vi "Main.GUI.vi"() -> ()   [LabVIEW 2015, in "Main.GUI.lvlib"]
uses:
  Main.GUI.lvlib
  Types/Multihead.StateVariables.ctl
  Types/TestStandGUI.Refs.ctl
  <vilib>/NI Veristand/Execution/Workspace/WorkspaceAPI.ctl
  <vilib>/NI Veristand/Execution/Workspace/SystemStateEventRef.ctl
  <vilib>/NI Veristand/Execution/Workspace/Target State Info.ctl
  <vilib>/NI Veristand/Execution/Workspace/Target State.ctl
  Execution GUI/Types/Execute.UserEventRefs.ctl
  <vilib>/NI Veristand/Execution/Workspace/SystemStateRegEventRef.ctl
  Analysis GUI/Types/Analysis.GUI.Parameters.ctl
  NationalInstruments.VeriStand
  <vilib>/NI/AMC/Read Termination Message.vi
  <vilib>/NI/AMC/Update Message Routing Info.vi
  <vilib>/NI/AMC/Create Multiple Messages.vi
  <vilib>/NI/AMC/Create Single Message.vi
  <vilib>/NI/AMC/Globals.vi
  <vilib>/NI/AMC/Send Message.vi
  <vilib>/NI Veristand/Execution/Workspace/NI VeriStand - Set Multiple Channel Values.vi
  <vilib>/NI/AMC/Queue Registry.vi
  <vilib>/NI/AMC/AMC.lvlib
  <vilib>/NI Veristand/Execution/Workspace/NI_VS Workspace ExecutionAPI.lvlib
  Execution GUI/Station.Execution.lvlib
  Analysis GUI/Analysis.lvlib
  NationalInstruments.VeriStand.ClientAPI
panel:
  in  "NIVS.Workspace Event":refnum<event-registration>
  in  "Application Manager":refnum<k7>(container)
  in  "SequenceFileView Manager":refnum<k7>(container)
  in  "ExecutionView Manager":refnum<k7>(container)
  in  "Tab Control":enum32{"TestStand", "GUIs"}(tab)
  in  "Entry Point 2 Button":refnum<k7>(container)
  in  "Open Sequence File Button":refnum<k7>(container)
  in  "Execution View":refnum<k7>(container)
  in  "Stop":bool
  out "Path":path
  in  "NIVS.Gateway IP Address":string="localhost"
  in  "Tree":string(tree)
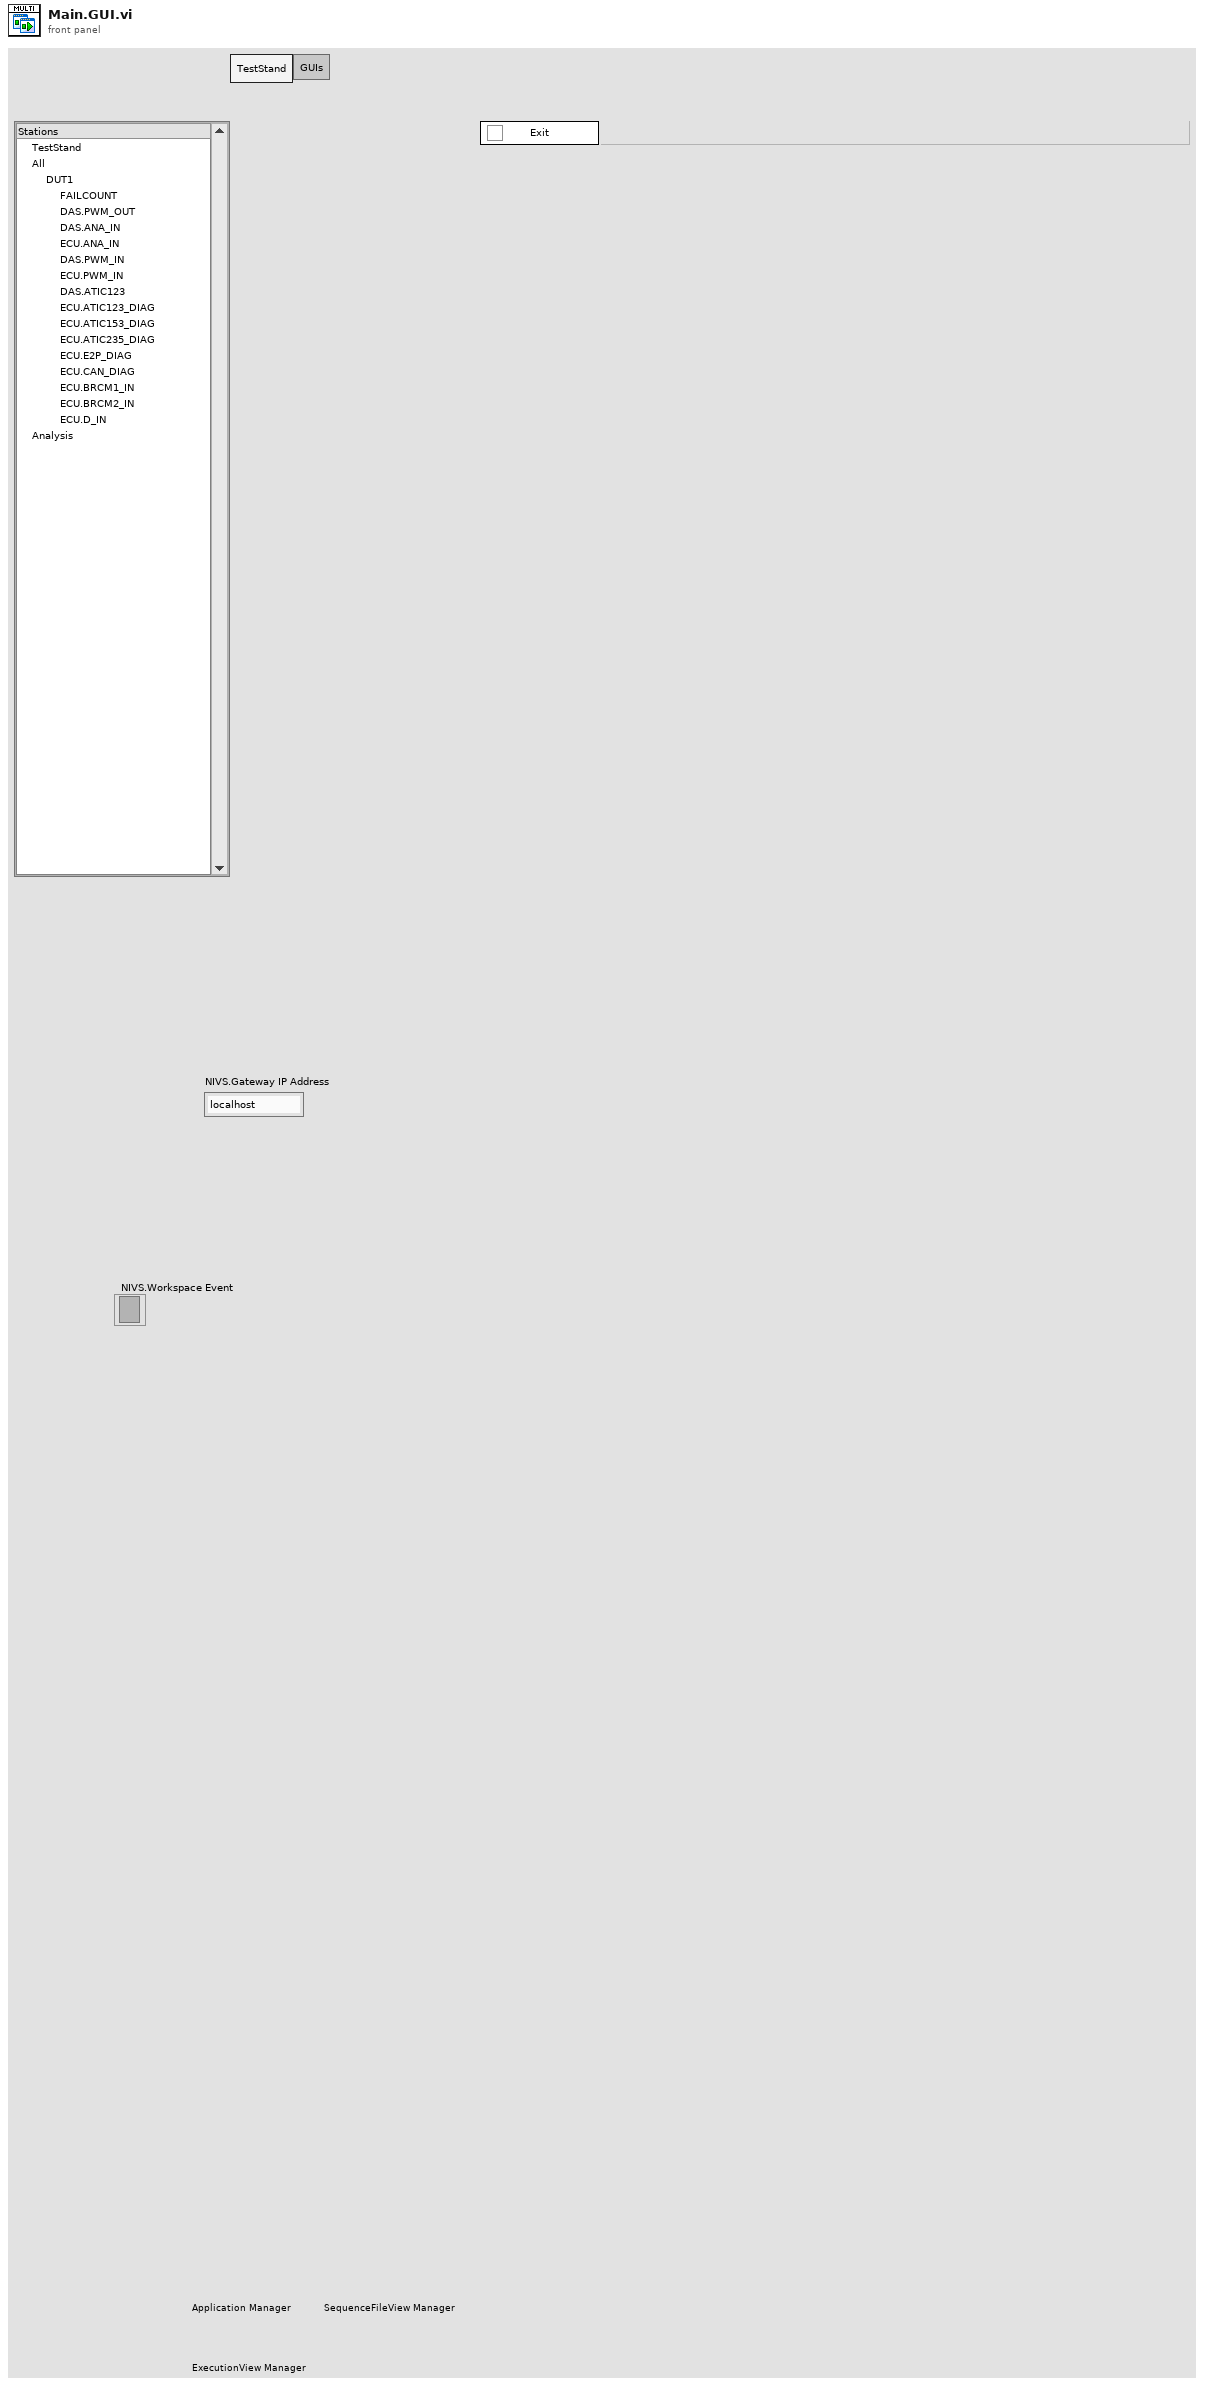
[diagram p1: front panel]
types:
  T1 = typedef "Main.GUI.lvlib/Multihead.StateVariables.ctl" = cluster{"DUTs.Name":string[], "Pages.Name":string[], "Pages.Ref":refnum<vi>[], "TS.UI":T2, "TS.Running":bool, "TS.Abort":bool, "NIVS.GatewayIPAddress":string, "NIVS.WorkspaceManager":T3, "NIVS.Open":bool, "NIVS.Deployed":bool, "NIVS.SystemStateRefs":T4, "NIVS.Events":T5, "UI.Tree":refnum<vi>, "UI.Path":refnum<vi>, "UI.Stop":refnum<vi>, "UI.Tab":refnum<vi>}
  T2 = typedef "Main.GUI.lvlib/TestStandGUI.Refs.ctl" = cluster{"References":cluster{"Event Callback":refnum<k27>, "Quit Application Event":refnum<user-event>, "Events":refnum<event-registration>, "Top level VI":refnum<vi>, "TestStand Engine":refnum<k7>, "Start Application Event":refnum<user-event>, "Stop Application Event":refnum<user-event>}, "Managers":cluster{"Application Manager":refnum<k7>, "SequenceFileView Manager":refnum<k7>, "ExecutionView Manager":refnum<k7>}, "Controls":cluster{"Execution View":refnum<k7>, "Run Button":refnum<k7>, "Open Button":refnum<k7>}}
  T3 = typedef "NI_VS Workspace ExecutionAPI.lvlib/WorkspaceAPI.ctl" = refnum<k24>
  T4 = typedef "NI_VS Workspace ExecutionAPI.lvlib/SystemStateEventRef.ctl" = cluster{"CustDatRef":refnum<user-event>, "EvtRef":refnum<k27>, "Target State User Event":refnum<user-event>}
  T5 = typedef "Station.Execution.lvlib/Execute.UserEventRefs.ctl" = cluster{"SystemChangeEvent":T6, "WorkspaceEvent":refnum<event-registration>}
  T6 = typedef "NI_VS Workspace ExecutionAPI.lvlib/SystemStateRegEventRef.ctl" = refnum<event-registration>
  T7 = typedef "AMC.lvlib/Message Queue.ctl" = refnum<queue>
  T8 = typedef "Analysis.lvlib/Analysis.GUI.Parameters.ctl" = cluster{"Results Path":path, "Temp Path":path, "Remote Path":path, "Analysis VIs":path[], "Report Passed?":bool, "Group Channels?":bool}
  T9 = cluster{"SystemChangeEvent":T6, "WorkspaceEvent":refnum<event-registration>, "Events":refnum<event-registration>}
  T10 = typedef "NI_VS Workspace ExecutionAPI.lvlib/SystemState.ctl" = u8
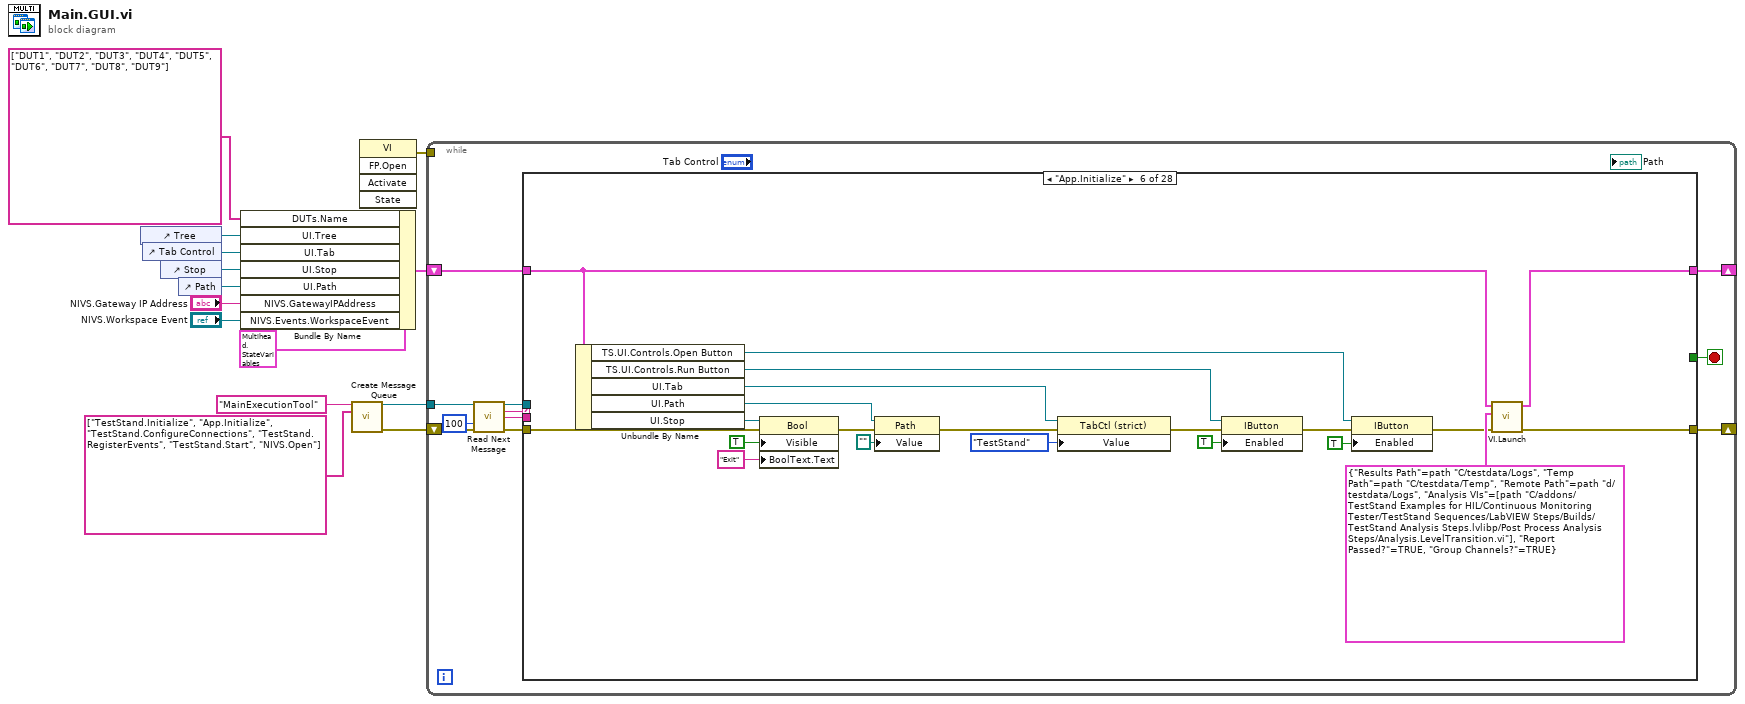
[diagram p0: block diagram]
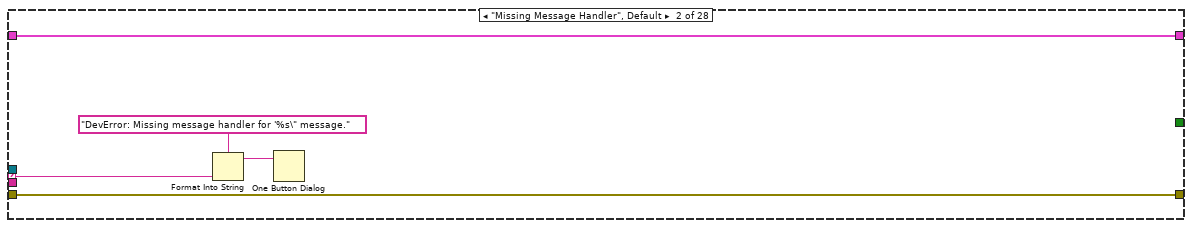
[diagram p3: hidden frame]
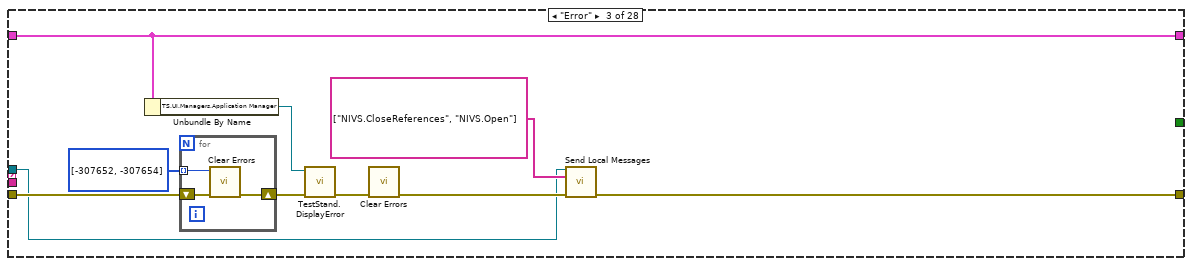
[diagram p4: hidden frame]
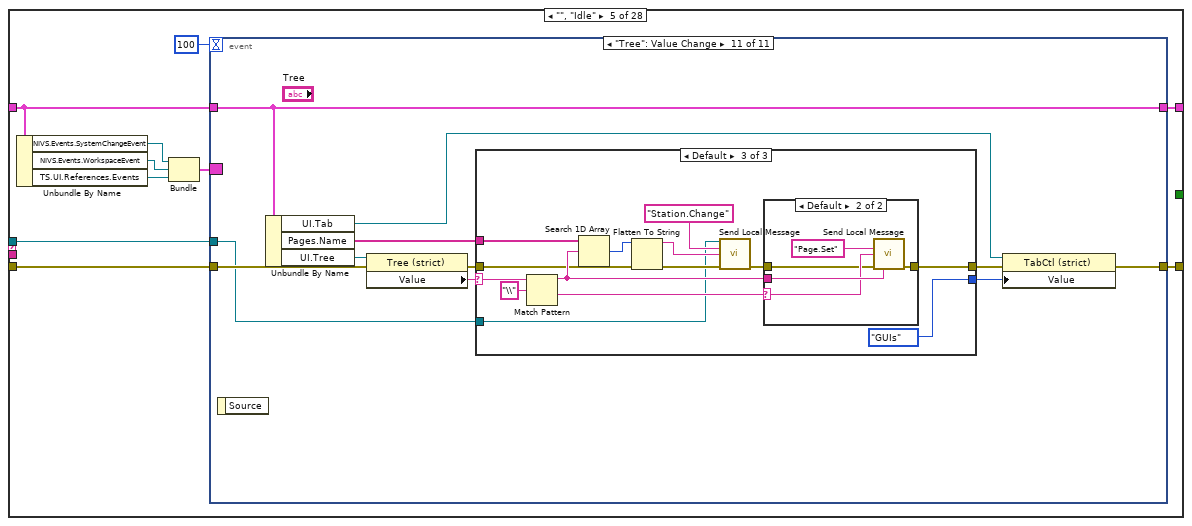
[diagram p6: hidden frame]
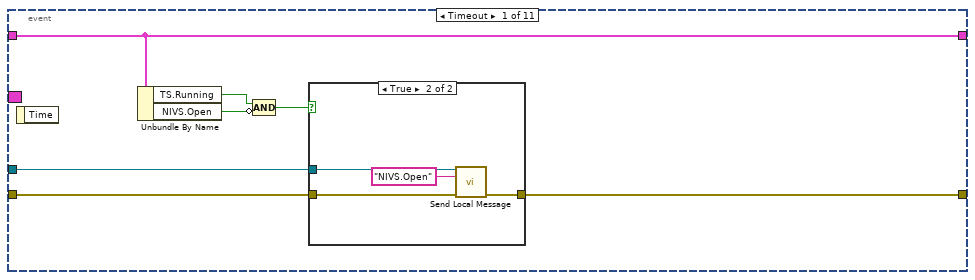
[diagram p7: hidden frame]
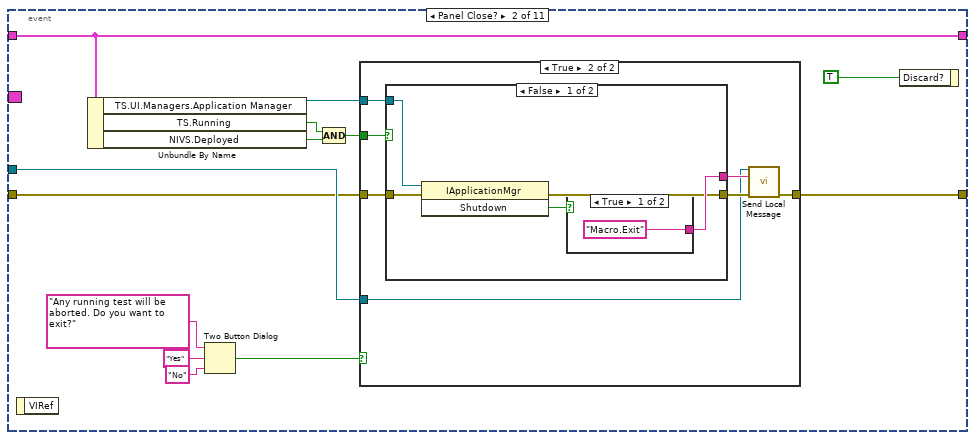
[diagram p9: hidden frame]
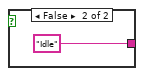
[diagram p11: hidden frame]
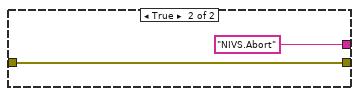
[diagram p12: hidden frame]
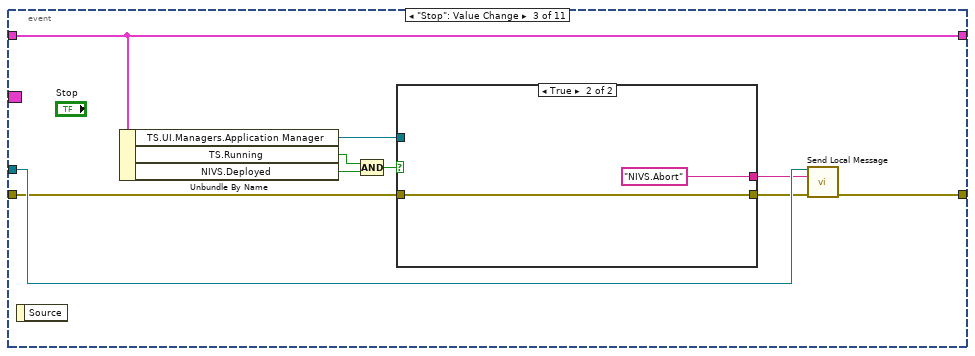
[diagram p13: hidden frame]
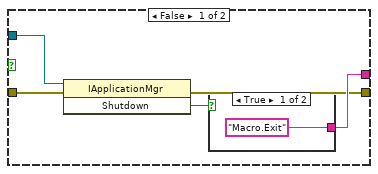
[diagram p14: hidden frame]
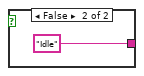
[diagram p15: hidden frame]
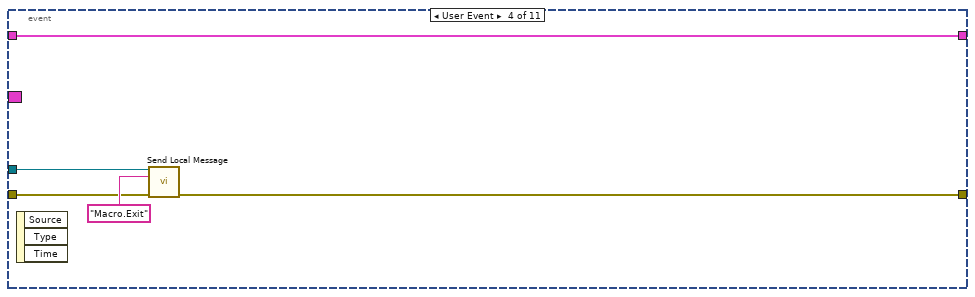
[diagram p16: hidden frame]
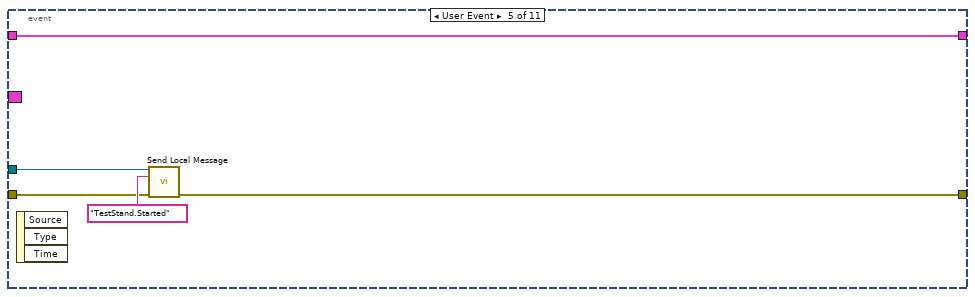
[diagram p17: hidden frame]
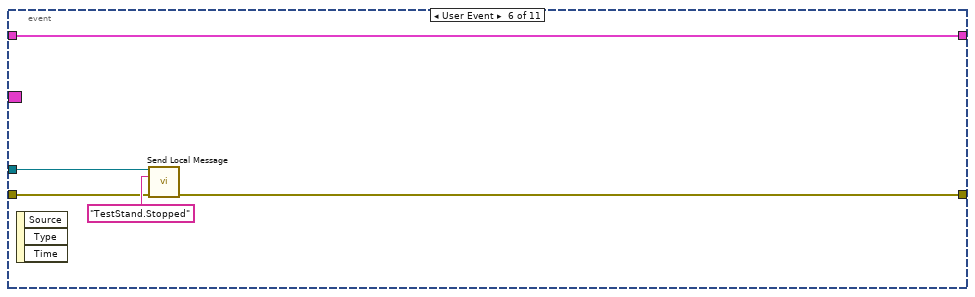
[diagram p18: hidden frame]
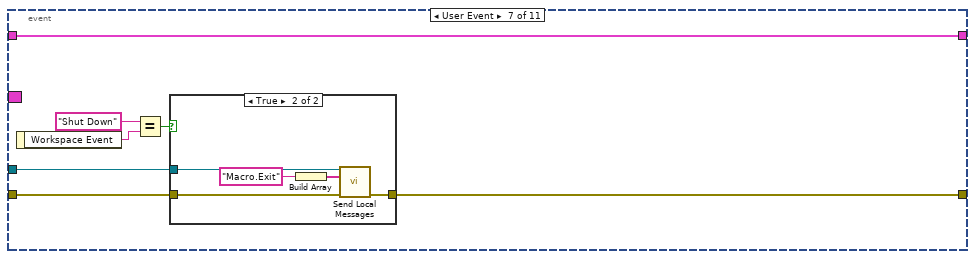
[diagram p19: hidden frame]
diagram:
  n1 = control-ref of="Tree"() -> (w13:refnum<vi>)
  n2 = control-ref of="Tab Control"() -> (w8:refnum<vi>)
  n3 = control-ref of="Stop"() -> (w7:refnum<vi>)
  n4 = control-ref of="Path"() -> (w1:refnum<vi>)
  n5 = Bundle By Name(cluster=T1 {"DUTs.Name"=[], "Pages.Name"=[], "Pages.Ref"=[], "TS.UI"={"References"={"Event Callback"=refnum, "Quit Application Event"=refnum, "Events"=refnum, "Top level VI"=refnum, "TestStand Engine"=refnum, "Start Application Event"=refnum, "Stop Application Event"=refnum}, "Managers"={"Application Manager"=refnum, "SequenceFileView Manager"=refnum, "ExecutionView Manager"=refnum}, "Controls"={"Execution View"=refnum, "Run Button"=refnum, "Open Button"=refnum}}, "TS.Running"=FALSE, "TS.Abort"=FALSE, "NIVS.GatewayIPAddress"="", "NIVS.WorkspaceManager"=refnum, "NIVS.Open"=FALSE, "NIVS.Deployed"=FALSE, "NIVS.SystemStateRefs"={"CustDatRef"=refnum, "EvtRef"=refnum, "Target State User Event"=refnum}, "NIVS.Events"={"SystemChangeEvent"=refnum, "WorkspaceEvent"=refnum}, "UI.Tree"=refnum, "UI.Path"=refnum, "UI.Stop"=refnum, "UI.Tab"=refnum} ("state variables in"), "DUTs.Name"=string[] ["DUT1", "DUT2", "DUT3", "DUT4", "DUT5", "DUT6", "DUT7", "DUT8", "DUT9"] ("All Tags"), "UI.Tree"=w13, "UI.Tab"=w8, "UI.Stop"=w7, "UI.Path"=w1, "NIVS.GatewayIPAddress"="NIVS.Gateway IP Address", "NIVS.Events.WorkspaceEvent"="NIVS.Workspace Event") -> (w5:T1)
  n6 = call <vilib>:"Create Message Queue.vi"("message queue name"="MainExecutionTool", "initial message names"=string[] ["TestStand.Initialize", "App.Initialize", "TestStand.ConfigureConnections", "TestStand.RegisterEvents", "TestStand.Start", "NIVS.Open"]) -> ("message queue out"=w3:T7, "error out"=w4:errorcluster)  [unwired: 12 in]
  n7 = invoke class="VI" method="FP.Open"() -> (error out=w2:errorcluster)  [unwired: 5 in, 4 out]
  n8 = while {
    shift-left: w4 -> [w15]
    shift-right: [w23] -> _
    tunnel: w3 -> [w21]
    shift-left: w5 -> [w25]
    shift-right: [w24] -> _
    tunnel: w2 -> [_]
    stop <- w16 stop-if-true
    n9 = call <vilib>:"Read Next Message.vi"("message queue in"=w21, "timeout (1 ms)"=100 ("Timeout"), "error in"=w15) -> ("message queue out"=w22:T7, "message name"=w19:string, "message value"=w18:string, "error out"=w20:errorcluster)  [unwired: 5 in, 4 out]
    n10 = case shown="\"App.Initialize\"" w19 {
      selector: w19 -> [_ w30 _ _ _ _ _ _ _ _ _ _ _ _ _ _ _ _ _ _ _ _ _ _ _ _ _ _]
      tunnel: [w27 w32 w41 w47 w53 w292 w301 w308 w317 w318 w350 w381 w394 w410 w421 w428 w463 w474 w489 w501 w513 w518 w538 w551 w554 w558 w562 w564] -> w24
      tunnel: w25 -> [w27 w32 w41 w47 w54 w293 w302 w308 w317 w320 w351 w381 w395 w410 w421 w428 w464 w474 w488 w501 w514 w519 w539 w552 w554 w558 w562 w564]
      tunnel: w22 -> [_ _ w34 _ w52 _ _ _ w315 w321 w347 _ _ _ _ _ _ _ _ _ _ _ w524 _ w555 _ _ _]
      tunnel: w20 -> [w26 w31 w38 w46 w57 w297 w306 w309 w316 w323 w352 w374 w396 w411 w420 _ w462 w475 w491 w502 w516 w522 w541 w549 w557 w559 w561 w563]
      tunnel: [w26 w31 w33 w46 w56 w294 w305 w309 w314 w322 w348 w370 w396 w407 w419 w429 w471 w472 w490 w500 w504 w521 w525 w548 w556 w559 w561 w563] -> w23
      tunnel: w18 -> [_ _ _ _ _ _ _ _ _ _ _ _ _ w408 w422 _ _ _ _ _ _ _ _ _ _ _ _ _]
      tunnel: [_ _ _ _ _ _ _ _ TRUE _ _ _ _ _ _ _ _ _ _ _ _ _ _ _ _ _ _ _] -> w16
      frame "---------- Framework Operations ----------" {
      }
      frame "Missing Message Handler", Default {
        n11 = Format Into String(format string="DevError: Missing message handler for '%s\" message." ("message"), w30) -> (resulting string=w28:string)  [unwired: 2 in, 1 out]
        n12 = One Button Dialog(message=w28) -> ()  [unwired: 2 out]
      }
      frame "Error" {
        n13 = Unbundle By Name(w41) -> ("TS.UI.Managers.Application Manager"=w42:refnum<k7>)
        n14 = for {
          shift-right: [w44] -> w37
          shift-left: w38 -> [w45]
          tunnel: i32[] [-307652, -307654] -> [w43] mode=indexing
          n15 = call <vilib>:"Clear Errors.vi"("error in (no error)"=w45, "specific error code to clear (0: all)"=w43) -> ("error out"=w44:errorcluster)  [unwired: 4 in, 1 out]
        }
        n16 = call "TestStand.DisplayError.vi"("error in (no error)"=w37, "Application Manager"=w42) -> ("error out"=w36:errorcluster)  [unwired: 9 out]
        n17 = call <vilib>:"Clear Errors.vi"("error in (no error)"=w36) -> ("error out"=w35:errorcluster)  [unwired: 5 in, 1 out]
        n18 = call <vilib>:"Send Local Messages.vi"("message queue in"=w34, "message names"=string[] ["NIVS.CloseReferences", "NIVS.Open"], "error in"=w35) -> ("error out"=w33:errorcluster)  [unwired: 10 in, 2 out]
      }
      frame "---------- Application Operations ----------" {
      }
      frame "", "Idle" {
        n19 = Unbundle By Name(w54) -> ("NIVS.Events.SystemChangeEvent"=w48:T6, "NIVS.Events.WorkspaceEvent"=w49:refnum<event-registration>, "TS.UI.References.Events"=w51:refnum<event-registration>)
        n20 = Bundle("SystemChangeEvent"=w48, "WorkspaceEvent"=w49, "Events"=w51) -> (w50:T9)  [unwired: 1 in]
        n21 = event shown="[10] \"Tree\": Value Change" {
          selector: w50 -> [_ _ _ _ _ _ _ _ _ _ _]
          dyn-events: _ -> [_ _ _ _ _ _ _ _ _ _ _]
          timeout: 100 -> [_ _ _ _ _ _ _ _ _ _ _]
          tunnel: w52 -> [w64 w80 w109 w122 w127 w132 w135 w151 w170 _ w248]
          tunnel: w57 -> [w63 w75 w102 w121 w126 w131 w136 w152 w168 w220 w250]
          tunnel: [w62 w81 w108 w120 w125 w130 w134 w150 w167 w219 w246] -> w56
          tunnel: w54 -> [w61 w74 w103 w119 w124 w129 w140 w148 w166 w224 w249]
          tunnel: [w61 w74 w103 w119 w124 w129 w140 w147 w165 w224 w249] -> w53
          event Timeout {
            n22 = event-data() -> ()  [unwired: 2 out]
            n23 = Unbundle By Name(w61) -> ("TS.Running"=w60:bool, "NIVS.Open"=w59:bool)
            n24 = Compound Arithmetic op=AND(w60, invert w59) -> (w58:bool)
            n25 = case shown="True" w58 {
              tunnel: w64 -> [_ w68]
              tunnel: w63 -> [w65 w67]
              tunnel: [w65 w66] -> w62
              frame False {
              }
              frame True {
                n26 = call <vilib>:"Send Local Message.vi"("message queue in"=w68, "message name"="NIVS.Open", "error in"=w67) -> ("error out"=w66:errorcluster)  [unwired: 10 in, 2 out]
              }
            }
          }
          event Panel Close? {
            n27 = event-data() -> ()  [unwired: 2 out]
            n28 = Unbundle By Name(w74) -> ("TS.UI.Managers.Application Manager"=w76:refnum<k7>, "TS.Running"=w79:bool, "NIVS.Deployed"=w78:bool)
            n29 = Two Button Dialog(message="Any running test will be aborted. Do you want to exit?", 1:"No" ("F button name (\"Cancel\")"), 2:"Yes" ("T button name (\"OK\")")) -> (T button?=w70:bool)
            n30 = Compound Arithmetic op=AND(w79, w78) -> (w77:bool)
            n31 = case shown="True" w70 {
              tunnel: [w83 w88] -> w81
              tunnel: w80 -> [_ w87]
              tunnel: w77 -> [_ w86]
              tunnel: w76 -> [_ w85]
              tunnel: w75 -> [w83 w84]
              frame False {
              }
              frame True {
                n32 = case shown="False" w86 {
                  tunnel: [w95 "NIVS.Abort"] -> w90
                  tunnel: [w94 w98] -> w89
                  tunnel: w85 -> [w93 _]
                  tunnel: w84 -> [w91 w98]
                  frame False {
                    n33 = invoke class="IApplicationMgr" method="Shutdown"(reference=w93, error in=w91) -> (error out=w94:errorcluster, "Shutdown"=w92:bool)  [unwired: 1 in, 1 out]
                    n34 = case shown="True" w92 {
                      tunnel: ["Macro.Exit" "Idle"] -> w95
                      frame True {
                      }
                      frame False {
                      }
                    }
                  }
                  frame True {
                  }
                }
                n35 = call <vilib>:"Send Local Message.vi"("message queue in"=w87, "message name"=w90, "error in"=w89) -> ("error out"=w88:errorcluster)  [unwired: 10 in, 2 out]
              }
            }
            n36 = event-data("Discard?"=TRUE) -> ()  [unwired: 1 in, 1 out]
          }
          event "Stop": Value Change {
            n37 = event-data() -> ()  [unwired: 2 out]
            n38 = Unbundle By Name(w103) -> ("TS.UI.Managers.Application Manager"=w104:refnum<k7>, "TS.Running"=w107:bool, "NIVS.Deployed"=w106:bool)
            n39 = Compound Arithmetic op=AND(w107, w106) -> (w105:bool)
            n40 = case shown="True" w105 {
              tunnel: [w114 "NIVS.Abort"] -> w100
              tunnel: [w113 w117] -> w101
              tunnel: w104 -> [w112 _]
              tunnel: w102 -> [w110 w117]
              frame False {
                n41 = invoke class="IApplicationMgr" method="Shutdown"(reference=w112, error in=w110) -> (error out=w113:errorcluster, "Shutdown"=w111:bool)  [unwired: 1 in, 1 out]
                n42 = case shown="True" w111 {
                  tunnel: ["Macro.Exit" "Idle"] -> w114
                  frame True {
                  }
                  frame False {
                  }
                }
              }
              frame True {
              }
            }
            n43 = call <vilib>:"Send Local Message.vi"("message queue in"=w109, "message name"=w100, "error in"=w101) -> ("error out"=w108:errorcluster)  [unwired: 10 in, 2 out]
          }
          event User Event {
            n44 = event-data() -> ()  [unwired: 4 out]
            n45 = call <vilib>:"Send Local Message.vi"("message queue in"=w122, "message name"="Macro.Exit", "error in"=w121) -> ("error out"=w120:errorcluster)  [unwired: 10 in, 2 out]
          }
          event User Event {
            n46 = event-data() -> ()  [unwired: 4 out]
            n47 = call <vilib>:"Send Local Message.vi"("message queue in"=w127, "message name"="TestStand.Started", "error in"=w126) -> ("error out"=w125:errorcluster)  [unwired: 10 in, 2 out]
          }
          event User Event {
            n48 = event-data() -> ()  [unwired: 4 out]
            n49 = call <vilib>:"Send Local Message.vi"("message queue in"=w132, "message name"="TestStand.Stopped", "error in"=w131) -> ("error out"=w130:errorcluster)  [unwired: 10 in, 2 out]
          }
          event User Event {
            n50 = event-data() -> ("Workspace Event"=w137:string)  [unwired: 1 out]
            n51 = Equal?(x="Shut Down" ("y"), y=w137) -> (x = y?=w139:bool)
            n52 = case shown="True" w139 {
              tunnel: w136 -> [w141 w146]
              tunnel: [w141 w145] -> w134
              tunnel: w135 -> [_ w144]
              frame False {
              }
              frame True {
                n53 = Build Array("Macro.Exit" ("y")) -> (w143:string[])
                n54 = call <vilib>:"Send Local Messages.vi"("message queue in"=w144, "message names"=w143, "error in"=w146) -> ("error out"=w145:errorcluster)  [unwired: 10 in, 2 out]
              }
            }
          }
          event User Event {
            n55 = event-data() -> ("SystemStateChange"=w149:string)  [unwired: 1 out]
            n56 = case shown="Default" w149 {
              tunnel: w152 -> [w158 w163]
              tunnel: w151 -> [w157 w162]
              tunnel: [w156 w161] -> w150
              tunnel: w148 -> [w155 w160]
              tunnel: [w154 w160] -> w147
              frame "Shut Down" {
                w153 = FALSE ("NIVS.Open")
                n57 = Bundle By Name(cluster=w155, "NIVS.Deployed"=w153, "NIVS.Open"=w153) -> (w154:T1)
                n58 = call <vilib>:"Send Local Messages.vi"("message queue in"=w157, "message names"=string[] ["NIVS.CloseReferences"], "error in"=w158) -> ("error out"=w156:errorcluster)  [unwired: 10 in, 2 out]
              }
              frame Default {
                n59 = call <vilib>:"Send Local Messages.vi"("message queue in"=w162, "message names"=string[] ["NIVS.CheckDeployment"], "error in"=w163) -> ("error out"=w161:errorcluster)  [unwired: 10 in, 2 out]
              }
            }
          }
          event Menu Selection (User) {
            n60 = event-data() -> ("ItemTag"=w169:string)  [unwired: 1 out]
            n61 = case shown="\"Macro.Exit\"" w169 {
              selector: w169 -> [_ w214]
              tunnel: w170 -> [w175 w210]
              tunnel: w168 -> [w177 w213]
              tunnel: [w178 w211] -> w167
              tunnel: w166 -> [w174 w209]
              tunnel: [w174 w209] -> w165
              frame "Macro.Exit" {
                n62 = Unbundle By Name(w174) -> ("TS.UI.Managers.Application Manager"=w173:refnum<k7>, "TS.Running"=w171:bool, "NIVS.Deployed"=w172:bool)
                n63 = Two Button Dialog(message="Any running test will be aborted. Do you want to exit?", 1:"No" ("F button name (\"Cancel\")"), 2:"Yes" ("T button name (\"OK\")")) -> (T button?=w179:bool)
                n64 = Compound Arithmetic op=AND(w171, w172) -> (w176:bool)
                n65 = case shown="True" w179 {
                  tunnel: [w183 w189] -> w178
                  tunnel: w175 -> [_ w188]
                  tunnel: w176 -> [_ w187]
                  tunnel: w173 -> [_ w186]
                  tunnel: w177 -> [w183 w185]
                  tunnel: w171 -> [_ w184]
                  frame False {
                  }
                  frame True {
                    n66 = case shown="False" w187 {
                      tunnel: [w196 "NIVS.Abort"] -> w191
                      tunnel: [w195 w206] -> w190
                      tunnel: w186 -> [w194 _]
                      tunnel: w185 -> [w193 w206]
                      tunnel: w184 -> [w192 _]
                      frame False {
                        n67 = case shown="False" w192 {
                          tunnel: [w201 "TestStand.Abort"] -> w196
                          tunnel: [w200 w205] -> w195
                          tunnel: w194 -> [w199 _]
                          tunnel: w193 -> [w197 w205]
                          frame False {
                            n68 = invoke class="IApplicationMgr" method="Shutdown"(reference=w199, error in=w197) -> (error out=w200:errorcluster, "Shutdown"=w198:bool)  [unwired: 1 in, 1 out]
                            n69 = case shown="True" w198 {
                              tunnel: ["Macro.Exit" "Idle"] -> w201
                              frame True {
                              }
                              frame False {
                              }
                            }
                          }
                          frame True {
                          }
                        }
                      }
                      frame True {
                      }
                    }
                    n70 = call <vilib>:"Send Local Message.vi"("message queue in"=w188, "message name"=w191, "error in"=w190) -> ("error out"=w189:errorcluster)  [unwired: 10 in, 2 out]
                  }
                }
              }
              frame Default {
                n71 = Unbundle By Name(w209) -> ("UI.Tree"=w208:refnum<vi>)
                n72 = property class="Tree (strict)"(reference=w208, error in=w213) -> (error out=w212:errorcluster, "Value"=w217:string)  [unwired: 1 out]
                n73 = Match Pattern(string=w217, regular expression="\\") -> (before substring=w215:string)  [unwired: 1 in, 3 out]
                n74 = call <vilib>:"Send Local Message.vi"("message queue in"=w210, "receiver process (\"\" - local)"=w215, "message name"=w214, "error in"=w212) -> ("error out"=w211:errorcluster)  [unwired: 9 in, 2 out]
              }
            }
          }
          event Menu Activation? {
            n75 = event-data() -> ("MenuRef"=w223:refnum<k9>)  [unwired: 1 out]
            n76 = Unbundle By Name(w224) -> ("TS.Abort"=w218:bool, "TS.Running"=w222:bool, "NIVS.Deployed"=w221:bool)
            n77 = case shown="True" w222 {
              tunnel: w223 -> [w229 w238]
              tunnel: w221 -> [_ w236]
              tunnel: [w225 w234] -> w219
              tunnel: w220 -> [w226 w233]
              tunnel: w218 -> [_ w232]
              frame False {
                n78 = Set Menu Item Info(7:"Macro.Exit" ("item tag"), 8:w226, 9:TRUE ("enabled"), 10:"Exit" ("item tag"), 11:w229) -> (0:w225:errorcluster)  [unwired: 2 in, 1 out]
              }
              frame True {
                n79 = case shown="False" w232 {
                  tunnel: w236 -> [w242 _]
                  tunnel: [w239 "Aborting..." ("item tag")] -> w235
                  frame False {
                    n80 = Select(t="Stop" ("item tag"), s=w242, f="Abort" ("item tag")) -> (s? t:f=w239:string)
                  }
                  frame True {
                  }
                }
                n81 = Not(x=w232) -> (.not. x?=w231:bool)
                n82 = Set Menu Item Info(7:"Macro.Exit" ("item tag"), 8:w233, 9:w231, 10:w235, 11:w238) -> (0:w234:errorcluster)  [unwired: 2 in, 1 out]
              }
            }
            n83 = event-data() -> ()  [unwired: 2 in, 1 out]
          }
          event "Tree": Value Change {
            n84 = event-data() -> ()  [unwired: 2 out]
            n85 = Unbundle By Name(w249) -> ("UI.Tab"=w245:refnum<vi>, "Pages.Name"=w253:string[], "UI.Tree"=w251:refnum<vi>)
            n86 = property class="Tree (strict)"(reference=w251, error in=w250) -> (error out=w252:errorcluster, "Value"=w254:string)  [unwired: 1 out]
            n87 = case shown="Default" w254 {
              selector: w254 -> [_ _ w260]
              tunnel: w252 -> [w256 w258 w266]
              tunnel: [w256 w258 w263] -> w247
              tunnel: w253 -> [_ _ w262]
              tunnel: w248 -> [_ _ w261]
              tunnel: [enum32{"TestStand", "GUIs"}."TestStand" ("Value") enum32{"TestStand", "GUIs"}."TestStand" ("Value") enum32{"TestStand", "GUIs"}."GUIs" ("Value")] -> w244
              frame "" {
              }
              frame "TestStand" {
              }
              frame Default {
                n88 = Match Pattern(string=w260, regular expression="\\") -> (before substring=w267:string, after substring=w268:string)  [unwired: 1 in, 2 out]
                n89 = Search 1D Array(1D array=w262, element=w267) -> (index of element=w270:i32)  [unwired: 1 in]
                n90 = Flatten To String(anything=w270, error in (no error)=w266) -> (data string=w269:string, error out=w265:errorcluster)  [unwired: 2 in, 1 out]
                n91 = call <vilib>:"Send Local Message.vi"("message queue in"=w261, "message name"="Station.Change", "message value"=w269, "error in"=w265) -> ("error out"=w264:errorcluster)  [unwired: 9 in, 2 out]
                n92 = case shown="Default" w268 {
                  selector: w268 -> [_ w277]
                  tunnel: w267 -> [_ w278]
                  tunnel: w264 -> [w273 w275]
                  tunnel: [w273 w274] -> w263
                  frame "" {
                  }
                  frame Default {
                    n93 = call <vilib>:"Send Local Message.vi"("receiver process (\"\" - local)"=w278, "message name"="Page.Set", "message value"=w277, "error in"=w275) -> ("error out"=w274:errorcluster)  [unwired: 9 in, 2 out]
                  }
                }
              }
            }
            n94 = property class="TabCtl (strict)"(reference=w245, error in=w247, "Value"=w244) -> (error out=w246:errorcluster)  [unwired: 1 out]
          }
        }
      }
      frame "App.Initialize" {
        n95 = Unbundle By Name(w293) -> ("TS.UI.Controls.Open Button"=w280:refnum<k7>, "TS.UI.Controls.Run Button"=w283:refnum<k7>, "UI.Tab"=w291:refnum<vi>, "UI.Path"=w296:refnum<vi>, "UI.Stop"=w298:refnum<vi>)
        n96 = property class="Bool"(reference=w298, error in=w297, "Visible"=TRUE, "BoolText.Text"="Exit" ("Boolean Text.Text")) -> (error out=w295:errorcluster)  [unwired: 1 out]
        n97 = property class="Path"(reference=w296, error in=w295, "Value"=path "") -> (error out=w290:errorcluster)  [unwired: 1 out]
        n98 = property class="TabCtl (strict)"(reference=w291, error in=w290, "Value"=enum32{"TestStand", "GUIs"}."TestStand") -> (error out=w284:errorcluster)  [unwired: 1 out]
        n99 = property class="IButton"(reference=w283, error in=w284, "Enabled"=TRUE) -> (error out=w282:errorcluster)  [unwired: 1 out]
        n100 = property class="IButton"(reference=w280, error in=w282, "Enabled"=TRUE) -> (error out=w281:errorcluster)  [unwired: 1 out]
        n101 = call "VI.Launch.vi"("error in (no error)"=w281, "Parameters"=T8 {"Results Path"=path "C:/testdata/Logs", "Temp Path"=path "C:/testdata/Temp", "Remote Path"=path "d:/testdata/Logs", "Analysis VIs"=[path "C:/addons/TestStand Examples for HIL/Continuous Monitoring Tester/TestStand Sequences/LabVIEW Steps/Builds/TestStand Analysis Steps.lvlibp/Post Process Analysis Steps/Analysis.LevelTransition.vi"], "Report Passed?"=TRUE, "Group Channels?"=TRUE}, "state variables"=w293) -> ("error out"=w294:errorcluster, "state variables"=w292:T1)  [unwired: 7 in]
      }
      frame "App.CreateEvents" {
        n102 = Unbundle By Name(w302) -> ("NIVS.WorkspaceManager"=w307:T3)
        n103 = call <vilib>:"NI VeriStand - Open Engine State Change Notification.vi"("error in (no error)"=w306, "WorkspaceManager in"=w307) -> ("error out"=w305:errorcluster, "SystemStateRefs"=w304:T4, "SystemChangeEventRef"=w303:T6, "WorkspaceManager out"=w300:T3)  [unwired: 6 in]
        n104 = Bundle By Name(cluster=w302, "NIVS.WorkspaceManager"=w300, "NIVS.Events.SystemChangeEvent"=w303, "NIVS.SystemStateRefs"=w304) -> (w301:T1)
      }
      frame "App.CloseReferences" {
        n105 = flat-sequence {
          tunnel: w308 -> [w312]
          tunnel: [w310] -> _
          frame #0 {
            n106 = Unbundle By Name(w312) -> ("Pages.Ref"=w311:refnum<vi>[])
            n107 = Close Reference(reference=w311) -> (error out=w310:errorcluster)  [unwired: 1 in]
          }
        }
      }
      frame "App.Exit" {
        n108 = call <vilib>:"Destroy Message Queue.vi"("message queue in"=w315, "error in"=w316) -> ("error out"=w314:errorcluster)  [unwired: 11 in, 2 out]
      }
      frame "NIVS.Open" {
        n109 = Unbundle By Name(w320) -> ("NIVS.GatewayIPAddress"=w319:string)
        n110 = case shown="No Error" w323 {
          selector: w323 -> [w326 w344]
          tunnel: w319 -> [w331 _]
          tunnel: [w325 w344] -> w322
          tunnel: w320 -> [w329 w345]
          tunnel: [w327 w345] -> w318
          tunnel: w321 -> [w324 _]
          frame No Error {
            n111 = call <vilib>:"NI VeriStand - Open Workspace Manager Reference.vi"("Gateway IP Address (\"\": localhost)"=w331) -> ("error out"=w330:errorcluster, "WorkspaceManager"=w328:T3)  [unwired: 9 in]
            n112 = case shown="No Error" w330 {
              tunnel: w329 -> [w339 w342]
              tunnel: w328 -> [w338 _]
              tunnel: [w336 w341] -> w327
              tunnel: w326 -> [w335 w343]
              tunnel: [w334 w343] -> w325
              tunnel: w324 -> [w333 _]
              frame No Error {
                n113 = Bundle By Name(cluster=w339, "NIVS.Open"=TRUE, "NIVS.WorkspaceManager"=w338) -> (w336:T1)
                n114 = call <vilib>:"Send Local Messages.vi"("message queue in"=w333, "message names"=string[] ["App.CreateEvents", "NIVS.CheckDeployment"], "error in"=w335) -> ("error out"=w334:errorcluster)  [unwired: 10 in, 2 out]
              }
              frame Error {
                n115 = Bundle By Name(cluster=w342, "NIVS.Open"=FALSE) -> (w341:T1)
              }
            }
          }
          frame Error {
          }
        }
      }
      frame "NIVS.CheckDeployment" {
        n116 = Unbundle By Name(w351) -> ("UI.Stop"=w346:refnum<vi>, "NIVS.WorkspaceManager"=w353:T3)
        n117 = call <vilib>:"NI VeriStand - Get System State.vi"("error in (no error)"=w352, "WorkspaceManager in"=w353) -> ("error out"=w349:errorcluster, "System State"=w354:T10)  [unwired: 5 in, 3 out]
        n118 = case shown="0, Default" w354 {
          tunnel: w351 -> [w361 w368]
          tunnel: [w360 w366] -> w350
          tunnel: w349 -> [w357 w364]
          tunnel: [w356 w363] -> w348
          tunnel: w347 -> [_ _]
          tunnel: w346 -> [w355 w365]
          frame 0, Default {
            # "Not connected"
            n119 = Bundle By Name(cluster=w361, "NIVS.Deployed"=FALSE ("Connected")) -> (w360:T1)
            n120 = property class="Bool"(reference=w355, error in=w357, "Visible"=FALSE) -> (error out=w356:errorcluster)  [unwired: 1 out]
          }
          frame 1 {
            # "Connected"
            n121 = property class="Bool"(reference=w365, error in=w364, "Visible"=TRUE) -> (error out=w363:errorcluster)  [unwired: 1 out]
            n122 = Bundle By Name(cluster=w368, "NIVS.Deployed"=TRUE ("Connected")) -> (w366:T1)
          }
        }
      }
      frame "NIVS.Abort" {
        n123 = Unbundle By Name(w381) -> ("UI.Stop"=w372:refnum<vi>, "NIVS.WorkspaceManager"=w373:T3)
        n124 = call <vilib>:"NI VeriStand - Get Alias List.vi"("error in (no error)"=w374, "WorkspaceManager in"=w373) -> ("error out"=w379:errorcluster, "Aliases"=w380:string[], "WorkspaceManager out"=w376:T3)  [unwired: 6 in, 1 out]
        n125 = for {
          tunnel: w380 -> [w392] mode=indexing
          tunnel: [w385] -> w377 mode=indexing if=w382
          shift-right: [w384] -> w378
          shift-left: w379 -> [w390]
          tunnel: [1.0] -> w375 mode=indexing if=w382
          n126 = Concatenate Strings("Aliases/" ("string"), w392) -> (w385:string)
          n127 = invoke class="StringArrayToNodePathUtils" method="NodePathToStringArray"(error in=w390, "nodePath"=w385) -> (error out=w384:errorcluster, "NodePathToStringArray"=w389:string[])  [unwired: 2 in, 2 out]
          n128 = Delete From Array(array=w389) -> (deleted portion=w388:string)  [unwired: 2 in, 1 out]
          n129 = To Upper Case(1:w388) -> (0:w387:string)
          n130 = Equal?(x="ABORT", y=w387) -> (x = y?=w382:bool)
        }
        n131 = call-poly <vilib>:"NI VeriStand - Set Channel Value.vi"("error in (no error)"=w378, "Values"=w375, "Channels"=w377, "WorkspaceManager in"=w376) -> ("error out"=w371:errorcluster)  [unwired: 6 in, 1 out]
        n132 = property class="Bool"(reference=w372, error in=w371, "BoolText.Text"="Stopping..." ("Boolean Text.Text")) -> (error out=w370:errorcluster)  [unwired: 1 out]
      }
      frame "NIVS.CloseReferences" {
        w393 = FALSE ("NIVS.Open")
        n133 = flat-sequence {
          tunnel: w395 -> [w400]
          tunnel: [w399] -> _
          tunnel: [w398] -> _
          tunnel: [w397] -> _
          frame #0 {
            n134 = Unbundle By Name(w400) -> ("NIVS.Events"=w401:T5, "NIVS.SystemStateRefs"=w403:T4, "NIVS.WorkspaceManager"=w402:T3)
            n135 = call <vilib>:"NI VeriStand - Close Workspace Manager Reference.vi"("WorkspaceManager"=w402) -> ("error out"=w397:errorcluster)  [unwired: 10 in]
            n136 = call <vilib>:"NI VeriStand - Close Engine State Change Notification.vi"("SystemStateRefs"=w403) -> ("error out"=w398:errorcluster)  [unwired: 10 in]
            n137 = Unregister For Events(event registration refnum=w401) -> (error out=w399:errorcluster)  [unwired: 1 in]
          }
        }
        n138 = Bundle By Name(cluster=w395, "NIVS.Open"=w393, "NIVS.Deployed"=w393) -> (w394:T1)
      }
      frame "Page.Published" {
        n139 = Unbundle By Name(w410) -> ("UI.Tab"=w405:refnum<vi>, "UI.Tree"=w412:refnum<vi>)
        n140 = property class="Tree (strict)"(reference=w412, error in=w411, "Value"=w408) -> (error out=w409:errorcluster)  [unwired: 1 out]
        n141 = case shown="\"\"" w408 {
          tunnel: w409 -> [w414 w416 w418]
          tunnel: [w414 w416 w418] -> w406
          tunnel: [enum32{"TestStand", "GUIs"}."TestStand" ("Value") enum32{"TestStand", "GUIs"}."TestStand" ("Value") enum32{"TestStand", "GUIs"}."GUIs" ("Value")] -> w404
          frame "" {
          }
          frame "TestStand" {
          }
          frame Default {
          }
        }
        n142 = property class="TabCtl (strict)"(reference=w405, error in=w406, "Value"=w404) -> (error out=w407:errorcluster)  [unwired: 1 out]
      }
      frame "Station.Change" {
        n143 = Unflatten From String(type=0 ("x-1"), binary string=w422, error in (no error)=w420) -> (value=w425:i32, error out=w427:errorcluster)  [unwired: 2 in, 1 out]
        n144 = Unbundle By Name(w421) -> ("Pages.Ref"=w423:refnum<vi>[])
        n145 = Index Array(array=w423, index=w425) -> (element=w426:refnum<vi>)
        n146 = invoke on="Sub Panel" class="SubPnl" method="Insert VI"(error in=w427, "VI Ref"=w426) -> (error out=w419:errorcluster)  [unwired: 2 in, 3 out]
      }
      frame "Processes.MacroExit" {
        w432 = "Macro.Exit"
        n147 = Unbundle By Name(w428) -> ("Pages.Name"=w430:string[])
        n148 = Delete From Array(array=w430, index=0) -> (deleted portion=w431:string, array with subset deleted=w441:string[])  [unwired: 1 in]
        n149 = call <vilib>:"Send Local Message.vi"("receiver process (\"\" - local)"=w431, "message name"=w432) -> ("error out"=w433:errorcluster)  [unwired: 11 in, 2 out]
        n150 = for {
          N: 50 -> [_]
          tunnel: w431 -> [w457]
          tunnel: w433 -> [w455]
          tunnel: [w454] -> w434
          stop <- w454 stop-if-true
          n151 = call <vilib>:"Get Queue From Registry.vi"("name"=w457, "error in"=w455) -> ("error out"=w454:errorcluster)  [unwired: 12 in, 1 out]
          n152 = Wait Until Next ms Multiple(millisecond multiple=u32 100) -> ()  [unwired: 1 out]
        }
        n153 = call <vilib>:"Clear Errors.vi"("error in (no error)"=w434) -> ("error out"=w435:errorcluster)  [unwired: 5 in, 1 out]
        n154 = for {
          tunnel: w441 -> [w451] mode=indexing
          tunnel: w432 -> [w452]
          tunnel: w435 -> [w453]
          tunnel: [w450] -> w437
          n155 = call <vilib>:"Send Local Message.vi"("receiver process (\"\" - local)"=w451, "message name"=w452, "error in"=w453) -> ("error out"=w450:errorcluster)  [unwired: 10 in, 2 out]
        }
        n156 = for {
          tunnel: w437 -> [w445]
          tunnel: 300 -> [w444]
          tunnel: w441 -> [w443] mode=indexing
          tunnel: [w442] -> w439
          n157 = for {
            N: w444 -> [_]
            tunnel: w443 -> [w449]
            tunnel: [w447] -> w442
            tunnel: w445 -> [w446]
            stop <- w447 stop-if-true
            n158 = call <vilib>:"Get Queue From Registry.vi"("name"=w449, "error in"=w446) -> ("error out"=w447:errorcluster)  [unwired: 12 in, 1 out]
            n159 = Wait Until Next ms Multiple(millisecond multiple=u32 100) -> ()  [unwired: 1 out]
          }
        }
        n160 = call <vilib>:"Clear Errors.vi"("error in (no error)"=w439) -> ("error out"=w429:errorcluster)  [unwired: 5 in, 1 out]
      }
      frame "TestStand.Initialize" {
        n161 = invoke class="IApplicationMgr" method="GetEngine"(reference="Application Manager", error in=w462) -> (reference out=w465:refnum<k7>, error out=w470:errorcluster, "GetEngine"=w459:refnum<k7>)  [unwired: 1 in]
        n162 = control-ref of="This VI"() -> (w466:refnum<vi>)
        n163 = Bundle By Name(cluster=w464, "TS.UI.References.Top level VI"=w466, "TS.UI.Managers.SequenceFileView Manager"="SequenceFileView Manager", "TS.UI.Managers.ExecutionView Manager"="ExecutionView Manager", "TS.UI.Controls.Execution View"="Execution View", "TS.UI.Controls.Run Button"="Entry Point 2 Button", "TS.UI.Controls.Open Button"="Open Sequence File Button", "TS.UI.Managers.Application Manager"=w465, "TS.UI.References.TestStand Engine"=w459) -> (w463:T1)
        n164 = call <vilib>:"TestStand - Set TestStand Application Window.vi"("error in (no error)"=w470, "Application Manager"=w465) -> ("error out"=w471:errorcluster)  [unwired: 1 in, 8 out]
      }
      frame "TestStand.ConfigureConnections" {
        n165 = Unbundle By Name(w474) -> ("TS.UI"=w473:T2)
        n166 = call "TestStand.ConnectCommands.vi"("error in"=w475, "TestStand.UI"=w473) -> ("error out"=w472:errorcluster)  [unwired: 9 in]
      }
      frame "TestStand.RegisterEvents" {
        w479 = cluster{"Number":i32} {"Number"=0}  # Stop Application Event
        w486 = cluster{"Number":i32} {"Number"=0}  # Start Application Event
        w499 = cluster{"Number":i32} {"Number"=0}  # Quit Application Event
        n167 = Create User Event(user event datatype=w499, error in=w491) -> (user event=w494:refnum<user-event>, error out=w487:errorcluster)
        n168 = Create User Event(user event datatype=w486, error in=w487) -> (user event=w484:refnum<user-event>, error out=w478:errorcluster)
        n169 = Create User Event(user event datatype=w479, error in=w478) -> (user event=w476:refnum<user-event>, error out=w477:errorcluster)
        n170 = register-events(error in=w477, w494, w484, w476) -> (reference out=w485:refnum<event-registration>, error out=w493:errorcluster)  [unwired: 1 in]
        n171 = Bundle By Name(cluster=w488, "TS.UI.References.Quit Application Event"=w494, "TS.UI.References.Start Application Event"=w484, "TS.UI.References.Stop Application Event"=w476, "TS.UI.References.Events"=w485) -> (w480:T1)
        n172 = Unbundle By Name(w480) -> ("TS.UI.Managers.Application Manager"=w482:refnum<k7>)
        n173 = vi-ref "TestStand.DisplaySequenceFileCallback.vi"() -> ("vi reference"=w497:refnum<vi>)
        n174 = vi-ref "TestStand.ExitApplicationCallback.vi"() -> ("vi reference"=w496:refnum<vi>)
        n175 = vi-ref "TestStand.DisplayExecutionCallback.vi"() -> ("vi reference"=w495:refnum<vi>)
        n176 = vi-ref "TestStand.ReportErrorCallback.vi"() -> ("vi reference"=w492:refnum<vi>)
        n177 = vi-ref "TestStand.SequenceOpenedCallback.vi"() -> ("vi reference"=w483:refnum<vi>)
        n178 = vi-ref "TestStand.EndExecutionCallback.vi"() -> ("vi reference"=w481:refnum<vi>)
        n179 = node(w493, w482, w497, w480, w482, w496, w480, w482, w495, w480, w482, w492, w480, w482, w483, w480, w482, w481, w480) -> (w498:refnum<k27>, w490:errorcluster)  [unwired: 1 in]
        n180 = Bundle By Name(cluster=w480, "TS.UI.References.Event Callback"=w498) -> (w489:T1)
      }
      frame "TestStand.Start" {
        n181 = Unbundle By Name(w501) -> ("TS.UI.Managers.Application Manager"=w503:refnum<k7>)
        n182 = invoke class="IApplicationMgr" method="Start"(reference=w503, error in=w502) -> (error out=w500:errorcluster)  [unwired: 1 in, 2 out]
      }
      frame "TestStand.Started" {
        n183 = Unbundle By Name(w514) -> ("TS.UI.Controls.Open Button"=w506:refnum<k7>, "TS.UI.Controls.Run Button"=w510:refnum<k7>, "UI.Stop"=w517:refnum<vi>)
        n184 = property class="Bool"(reference=w517, error in=w516, "Visible"=FALSE, "BoolText.Text"="Stop" ("Boolean Text.Text")) -> (error out=w509:errorcluster)  [unwired: 1 out]
        n185 = property class="IButton"(reference=w510, error in=w509, "Enabled"=FALSE) -> (error out=w505:errorcluster)  [unwired: 1 out]
        n186 = Bundle By Name(cluster=w514, "TS.Running"=TRUE) -> (w513:T1)
        n187 = property class="IButton"(reference=w506, error in=w505, "Enabled"=FALSE) -> (error out=w504:errorcluster)  [unwired: 1 out]
      }
      frame "TestStand.Abort" {
        n188 = Unbundle By Name(w519) -> ("TS.UI.References.TestStand Engine"=w523:refnum<k7>)
        n189 = invoke class="IEngine" method="TerminateAll"(reference=w523, error in=w522) -> (error out=w521:errorcluster)  [unwired: 1 in, 2 out]
        n190 = Bundle By Name(cluster=w519, "TS.Abort"=TRUE) -> (w518:T1)
      }
      frame "TestStand.Stopped" {
        n191 = Unbundle By Name(w539) -> ("TS.Abort"=w527:bool, "TS.UI.Managers.Application Manager"=w528:refnum<k7>, "TS.UI.Controls.Open Button"=w530:refnum<k7>, "TS.UI.Controls.Run Button"=w535:refnum<k7>, "UI.Stop"=w542:refnum<vi>)
        n192 = Bundle By Name(cluster=w539, "TS.Running"=FALSE) -> (w538:T1)
        n193 = property class="Bool"(reference=w542, error in=w541, "Visible"=TRUE, "BoolText.Text"="Exit" ("Boolean Text.Text")) -> (error out=w534:errorcluster)  [unwired: 1 out]
        n194 = property class="IButton"(reference=w535, error in=w534, "Enabled"=TRUE) -> (error out=w531:errorcluster)  [unwired: 1 out]
        n195 = property class="IButton"(reference=w530, error in=w531, "Enabled"=TRUE) -> (error out=w529:errorcluster)  [unwired: 1 out]
        n196 = invoke class="IApplicationMgr" method="CloseAllExecutions"(reference=w528, error in=w529) -> (error out=w526:errorcluster)  [unwired: 1 in, 2 out]
        n197 = case shown="True" w527 {
          tunnel: w526 -> [w543 w547]
          tunnel: [w543 w546] -> w525
          tunnel: w524 -> [_ w545]
          frame False {
          }
          frame True {
            n198 = call <vilib>:"Send Local Message.vi"("message queue in"=w545, "message name"="Macro.Exit", "error in"=w547) -> ("error out"=w546:errorcluster)  [unwired: 10 in, 2 out]
          }
        }
      }
      frame "TestStand.Shutdown" {
        n199 = call "TestStand.Shutdown.vi"("error in (no error)"=w549, "state variables in"=w552) -> ("error out"=w548:errorcluster)  [unwired: 9 in]
        n200 = Bundle By Name(cluster=w552, "TS.Running"=FALSE) -> (w551:T1)
      }
      frame "Macro.Exit" {
        n201 = call <vilib>:"Send Local Messages.vi"("message queue in"=w555, "message names"=string[] ["UI.SetBusy", "TestStand.Shutdown", "Processes.MacroExit", "NIVS.CloseReferences", "UI.UnsetBusy", "UI.Close", "App.CloseReferences", "App.Exit"], "error in"=w557) -> ("error out"=w556:errorcluster)  [unwired: 10 in, 2 out]
      }
      frame "UI.Close" {
        n202 = flat-sequence {
          tunnel: w558 -> [_]
          tunnel: [w560] -> _
          frame #0 {
            n203 = invoke class="VI" method="FP.Close"() -> (error out=w560:errorcluster)  [unwired: 3 in, 2 out]
          }
        }
      }
      frame "UI.SetBusy" {
        n204 = call <vilib>:"Set Busy.vi"() -> ()  [unwired: 10 in, 2 out]
      }
      frame "UI.UnsetBusy" {
        n205 = call <vilib>:"Unset Busy.vi"() -> ()  [unwired: 11 in, 1 out]
      }
    }
  }
